vi "Auto Setup.vi"(8 "error in (no error)":errorcluster, 11 "Agilent 3054A in":refnum<class "Agilent 3054A.lvclass">) -> (0 "error out":errorcluster, 3 "Agilent 3054A out":refnum<class "Agilent 3054A.lvclass">)   [LabVIEW 2016, in "Oscilloscope.lvlib" / "Agilent 3054A.lvclass"]
uses:
  Agilent 3054A.lvclass
  Agilent 3054A.lvclass/Agilent 3054A.ctl
  <instrlib>/Agilent 2000 3000 X-Series/Agilent 2000 3000 X-Series.lvlib
panel:
  in  "Channel":i32(ring) items=["Channel 1"=0, "Channel 2"=1, "Channel 3"=2, "Channel 4"=3, "Digital Bus Low"=9, "Digital Bus High"=10]
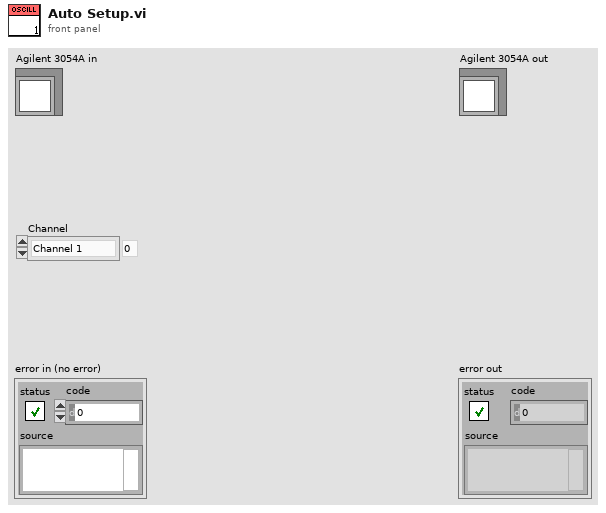
[diagram p1: front panel]
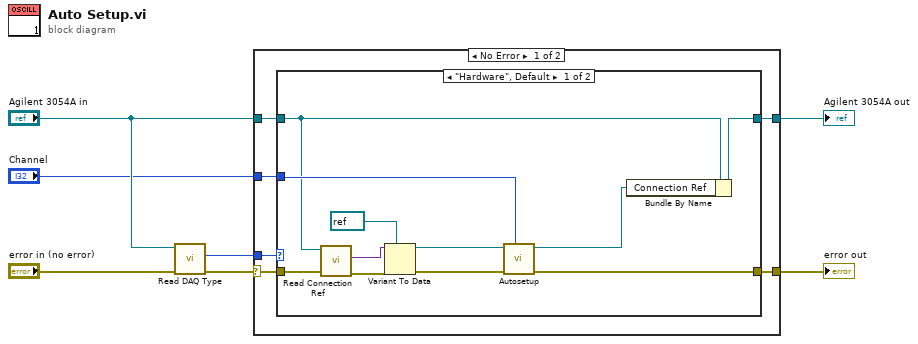
[diagram p0: block diagram]
diagram:
  n1 = call-dynamic "Read DAQ Type.vi"("error in (no error)"="error in (no error)", "Agilent 3054A in"="Agilent 3054A in") -> ("error out"=w6:errorcluster, "DAQ Type"=w5:enum16{"Hardware", "Simulation"})  [unwired: 7 in, 1 out]
  n2 = case shown="No Error" w6 {
    selector: w6 -> [w12 w27]
    tunnel: w5 -> [w13 _]
    tunnel: "Agilent 3054A in" -> [w11 w28]
    tunnel: "Channel" -> [w10 _]
    tunnel: [w9 w28] -> w2
    tunnel: [w8 w27] -> w1
    frame No Error {
      n3 = case shown="\"Hardware\", Default" w13 {
        tunnel: w12 -> [w24 w25]
        tunnel: w11 -> [w17 w26]
        tunnel: w10 -> [w18 _]
        tunnel: [w15 w26] -> w9
        tunnel: [w16 w25] -> w8
        frame "Hardware", Default {
          n4 = call-dynamic "Read Connection Ref.vi"("error in (no error)"=w24, "Agilent 3054A in"=w17) -> ("error out"=w23:errorcluster, "Connection Ref"=w22:variant)  [unwired: 7 in, 1 out]
          n5 = Variant To Data(error in=w23, type=refnum<visa-resource-name> refnum ("VISA resource name"), Variant=w22) -> (data=w20:refnum<visa-resource-name>, error out=w19:errorcluster)
          n6 = call <instrlib>:"Autosetup.vi"("Auto Scale Source (0: Channel 1)"=w18, "error in (no error)"=w19, "VISA resource name"=w20) -> ("error out"=w16:errorcluster, "VISA resource name out"=w14:refnum<visa-resource-name>)  [unwired: 7 in]
          n7 = Bundle By Name(cluster=w17, "Connection Ref"=w14) -> (w15:refnum<class "Agilent 3054A.lvclass">)
        }
        frame "Simulation" {
        }
      }
    }
    frame Error {
    }
  }
  "error out" <- w1
  "Agilent 3054A out" <- w2
